vi "niSwitch Attach to Session.vi"(7 "simulate (F)":bool, 8 "error in":errorcluster, 9 "reset device (T)":bool=TRUE, 10 "topology name":T1="Configured Topology", 11 "resource name":string) -> (0 "error out":errorcluster, 2 "session out":variant, 3 "session factory out":refnum<class "Session Factory.lvclass">)   [LabVIEW 2021, in "Session Management niSwitch.lvlib" / "Session Factory.lvclass"]
doc: "Attaches to an existing session of the provided <b>resource name</b>."
uses:
  Session Factory.lvclass
  <instrlib>/niSwitch/niSwitch.llb/niSwitch Topologies.ctl
  <vilib>/gRPC/Generated APIs/ni/measurementlink/discovery/v1/RPC Messages/ni_measurementlink_discovery_v1_ResolveServiceRequest.ctl
  <vilib>/Plug-In SDKs/Sessions/Instrument/ISession Factory/Session Initialization Parameters.ctl
  <vilib>/Plug-In SDKs/Sessions/Instrument/ISession Factory/Remote Connection Options.ctl
  <vilib>/Plug-In SDKs/Sessions/Instrument/ISession Factory/Initialize and Close Session Behavior.ctl
  <vilib>/Plug-In SDKs/Clients/Discovery V1/NI Discovery V1 Client.lvlib
  <vilib>/gRPC/Generated APIs/ni/measurementlink/discovery/v1/ni.measurementlink.discovery.v1.api.lvlib
  <vilib>/Plug-In SDKs/Sessions/Instrument/ISession Factory/ISession Factory.lvclass
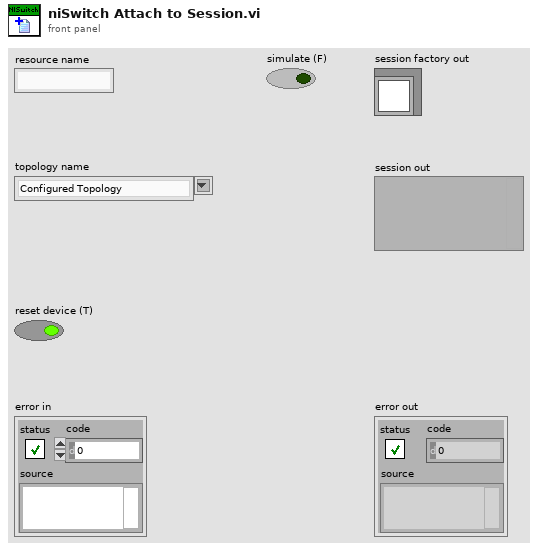
[diagram p1: front panel]
types:
  T1 = typedef "niSwitch Topologies.ctl" = string
  T2 = typedef "NI Session Management Instrument.lvlib/ISession Factory.lvclass/Initialize and Close Session Behavior.ctl" = enum16{"Initialize and Close", "Attach and Detach", "Initialize and Detach", "Attach and Close"}
  T3 = typedef "NI Session Management Instrument.lvlib/ISession Factory.lvclass/Remote Connection Options.ctl" = cluster{"session name":string, "address":string, "port":u32}
  T4 = typedef "NI Session Management Instrument.lvlib/ISession Factory.lvclass/Session Initialization Parameters.ctl" = cluster{"resource name":string, "session name":string}
  T5 = typedef "ni.measurementlink.discovery.v1.api.lvlib/ni_measurementlink_discovery_v1_ResolveServiceRequest.ctl" = cluster{"provided_interface":string, "service_class":string, "deployment_target":string, "version":string}
  T6 = typedef "ni.measurementlink.discovery.v1.api.lvlib/ni_measurementlink_discovery_v1_ServiceLocation.ctl" = cluster{"location":string, "insecure_port":string, "ssl_authenticated_port":string}
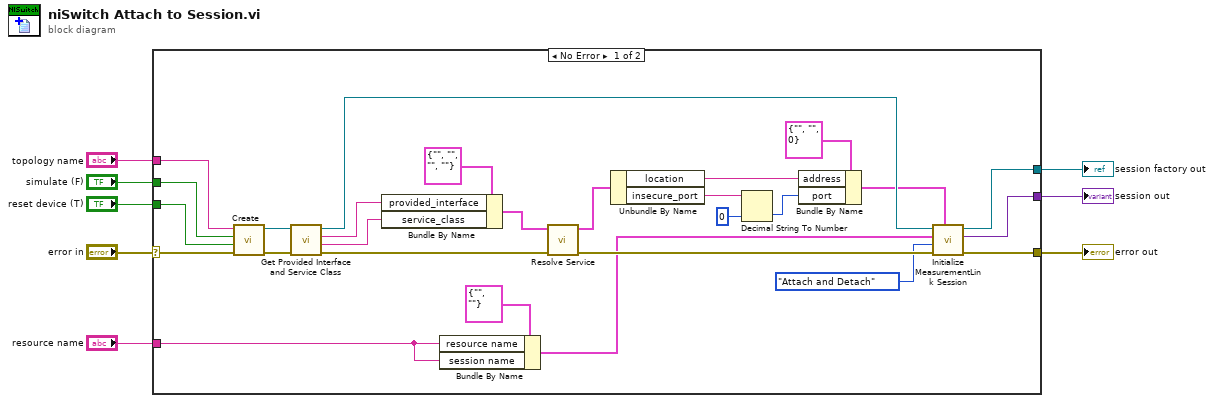
[diagram p0: block diagram]
diagram:
  n1 = case shown="No Error" "error in" {
    selector: "error in" -> [w31 w36]
    tunnel: [w22 w36] -> w1
    tunnel: "topology name" -> [w34 _]
    tunnel: "simulate (F)" -> [w33 _]
    tunnel: "reset device (T)" -> [w32 _]
    tunnel: [w20 _] -> w3
    tunnel: "resource name" -> [w9 _]
    tunnel: [w11 _] -> w2
    frame No Error {
      n2 = call "Create.vi"("error in"=w31, "reset device"=w32, "simulate"=w33, "topology name"=w34) -> ("error out"=w35:errorcluster, "session factory out"=w29:refnum<class "Session Factory.lvclass">)  [unwired: 6 in]
      n3 = call-dynamic "Get Provided Interface and Service Class.vi"("error in"=w35, "session factory in"=w29) -> ("error out"=w30:errorcluster, "service class"=w25:string, "provided interface"=w26:string, "session factory out"=w21:refnum<class "Session Factory.lvclass">)  [unwired: 6 in]
      n4 = Bundle By Name(cluster=T5 {"provided_interface"="", "service_class"="", "deployment_target"="", "version"=""} ("request data"), "provided_interface"=w26, "service_class"=w25) -> (w24:T5)
      n5 = Bundle By Name(cluster=T4 {"resource name"="", "session name"=""} ("session initialization parameters"), "resource name"=w9, "session name"=w9) -> (w12:T4)
      n6 = call <vilib>:"Resolve Service.vi"("error in"=w30, "request data"=w24) -> ("error out"=w28:errorcluster, "response data"=w23:T6)  [unwired: 8 in]
      n7 = Unbundle By Name(w23) -> ("location"=w14:string, "insecure_port"=w18:string)
      n8 = Decimal String To Number(string=w18, default (0L)=u32 0 ("default (0 I32)")) -> (number=w19:u32)  [unwired: 1 in, 1 out]
      n9 = Bundle By Name(cluster=T3 {"session name"="", "address"="", "port"=0} ("remote connection options"), "address"=w14, "port"=w19) -> (w16:T3)
      n10 = call-dynamic "Initialize MeasurementLink Session.vi"("remote connection options"=w16, "error in"=w28, "initialize and close session behavior"=Initialize_and_Close_Session_Behavior."Attach and Detach", "session initialization parameters"=w12, "session factory in"=w21) -> ("error out"=w22:errorcluster, "session out"=w11:variant, "session factory out"=w20:refnum<class "Session Factory.lvclass">)  [unwired: 4 in]
    }
    frame Error {
    }
  }
  "error out" <- w1
  "session factory out" <- w3
  "session out" <- w2
